vi "sub_addNextGuessToQueue.vi"(11 "queues":T1) -> (3 "no guesses left ?":bool)   [LabVIEW 2018]
uses:
  guess.ctl
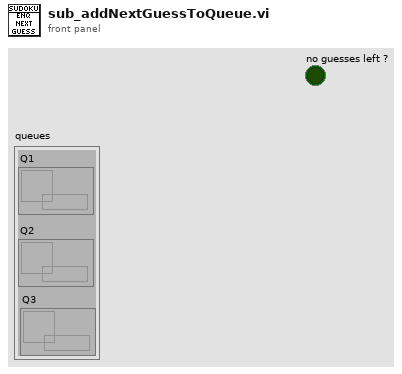
[diagram p1: front panel]
types:
  T1 = cluster{"Q1":refnum<queue>, "Q2":refnum<queue>, "Q3":refnum<queue>}
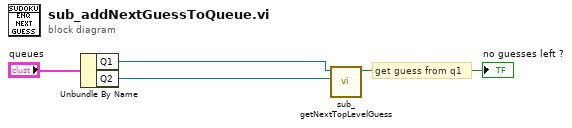
[diagram p0: block diagram]
diagram:
  # "get guess from q1"
  n1 = Unbundle By Name("queues") -> ("Q1"=w2:refnum<queue>, "Q2"=w1:refnum<queue>)
  n2 = call "sub_getNextTopLevelGuess.vi"("Q2"=w1, "Q1"=w2) -> ("q1 empty ?"=→"no guesses left ?":bool)  [unwired: 8 in, 1 out]
